vi "ALTS-2015 Get the order of OPC Registers.vi"(8 "error in (no error)":errorcluster, 9 "Register Names - Enum":string[](array[string]), 11 "Register Names - INI":string[](array[string])) -> (0 "error out":errorcluster, 3 "Channel Order":i32[](array[numeric]))   [LabVIEW 2013]
doc: "Copyright © 2005, Soliton Technologies.\nAll rights reserved."
uses:
  Controls/ALTS-2015 Mode Cases.ctl
  Instance           1 38Saved   Get the order of OPC Registers .vi
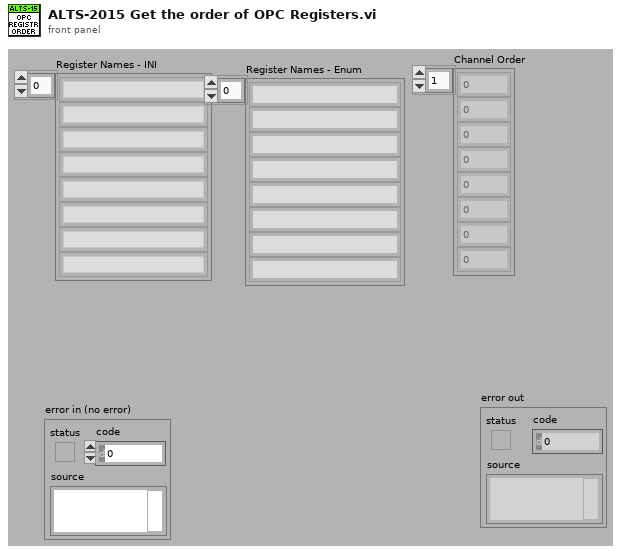
[diagram p1: front panel]
types:
  T1 = typedef "ALTS-2015 Mode Cases.ctl" = enum16{"Set Mode", "Read Mode"}
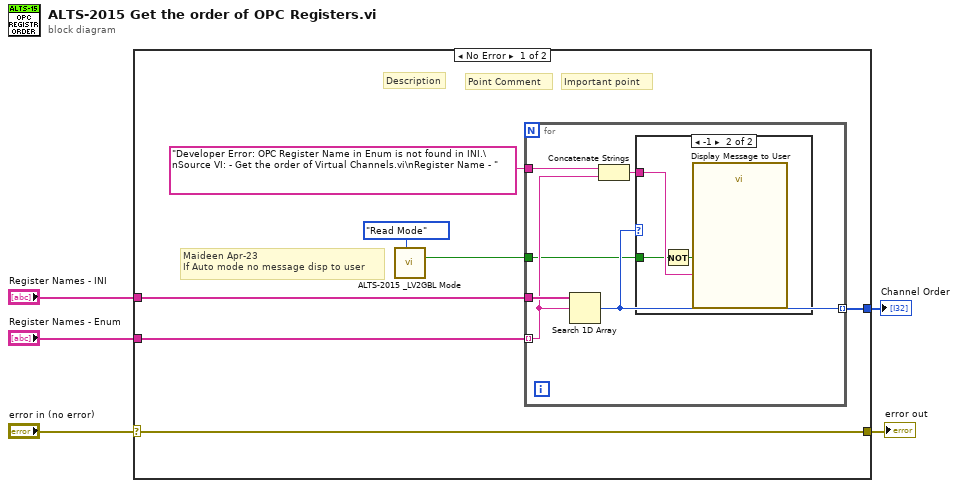
[diagram p0: block diagram]
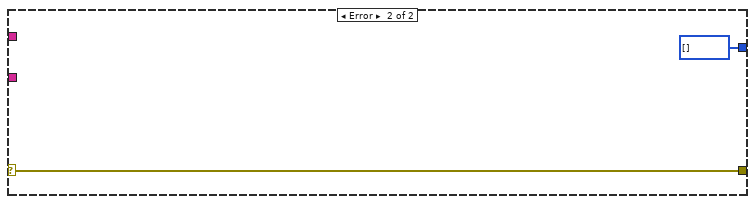
[diagram p3: hidden frame]
diagram:
  n1 = case shown="No Error" "error in (no error)" {
    selector: "error in (no error)" -> [w12 w23]
    tunnel: [w12 w23] -> w4
    tunnel: "Register Names - Enum" -> [w11 _]
    tunnel: "Register Names - INI" -> [w8 _]
    tunnel: [w9 i32[] []] -> w1
    frame No Error {
      # "Maideen Apr-23\nIf Auto mode no message disp to user"
      # "Point Comment"
      # "Important point"
      # "Description"
      n2 = call "ALTS-2015 _LV2GBL Mode.vi"("Options"=ALTS-2015_Mode_Cases."Read Mode") -> ("Auto mode?"=w6:bool)  [unwired: 9 in, 1 out]
      n3 = for {
        tunnel: w8 -> [w18]
        tunnel: w11 -> [w15] mode=indexing
        tunnel: [w17] -> w9 mode=indexing
        tunnel: "Developer Error: OPC Register Name in Enum is not found in INI.\nSource VI: - Get the order of Virtual Channels.vi\nRegister Name - " ("Virtual Channel Name") -> [w16]
        tunnel: w6 -> [w13]
        n4 = Search 1D Array(1D array=w18, element=w15) -> (index of element=w17:i32)  [unwired: 1 in]
        n5 = Concatenate Strings(w16, w15) -> (w14:string)
        n6 = case shown="-1" w17 {
          tunnel: w14 -> [_ w21]
          tunnel: w13 -> [_ w20]
          frame 0, Default {
          }
          frame -1 {
            n7 = Not(x=w20) -> (.not. x?=w19:bool)
            n8 = call "Display Message to User"("Enable"=w19, "Message"=w21) -> ()  [unwired: 8 in, 2 out]
          }
        }
      }
    }
    frame Error {
    }
  }
  "error out" <- w4
  "Channel Order" <- w1
